vi "unflattenTemperatureAbsFromXML_Array.vi"(8 "error in (no error)":errorcluster, 9 "temperatureAbsUnitInXML":T1, 10 "xmlString":string, 11 "temperatureAbsForType":dbl[unit][](array[numeric])=[273.41179938779914, 273.6735987755983, 273.93539816339745, 274.19719755119655]) -> (0 "error out":errorcluster, 3 "temperatureAbs":dbl[unit][](array[numeric]))   [LabVIEW 2012, in "UnitsAndXML.lvlib"]
uses:
  <userlib>/Common/UnitsAndXML/UnitsAndXML.lvlib
  <userlib>/Common/UnitsAndXML/FlattenItemWithUnitToXML/FlattenTemperatureAbsToXML/TemperatureAbsUnit.ctl
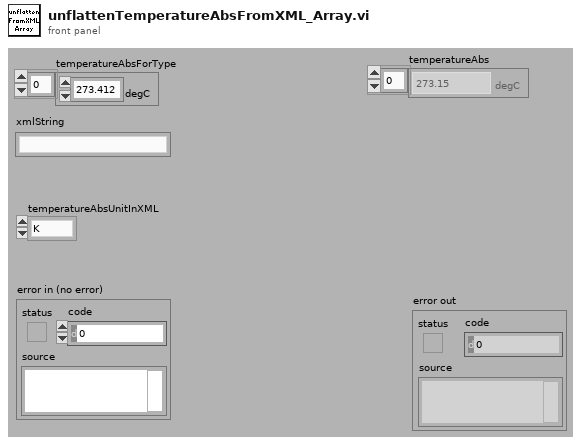
[diagram p1: front panel]
types:
  T1 = typedef "UnitsAndXML.lvlib/TemperatureAbsUnit.ctl" = enum16{"K", "degC", "degF"}
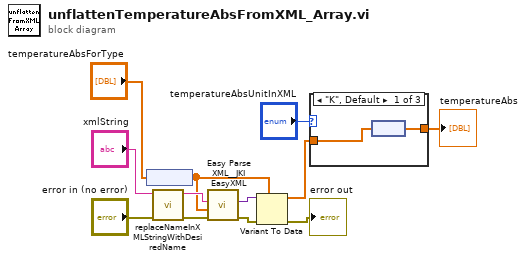
[diagram p0: block diagram]
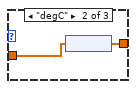
[diagram p2: hidden frame]
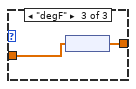
[diagram p3: hidden frame]
diagram:
  n1 = node("temperatureAbsForType") -> (w8:dbl[])
  n2 = call <userlib>:"replaceNameInXMLStringWithDesiredName.vi"("error in"="error in (no error)", "xmlString"="xmlString") -> ("error out"=w1:errorcluster, "revisedXMLString"=w9:string)  [unwired: 8 in]
  n3 = call <vilib>:"Easy Parse XML__JKI EasyXML.vi"("error in (no error)"=w1, "LabVIEW Data (Type)"=w8, "XML String"=w9) -> ("error out"=w4:errorcluster, "LabVIEW Data"=w11:variant)  [unwired: 7 in]
  n4 = Variant To Data(error in=w4, type=w8, Variant=w11) -> (data=w7:dbl[], error out=→"error out":errorcluster)
  n5 = case shown="\"K\", Default" "temperatureAbsUnitInXML" {
    tunnel: w7 -> [w13 w16 w18]
    tunnel: [w14 w15 w17] -> w6
    frame "K", Default {
      n6 = node(w13) -> (w14:dbl[unit][])
    }
    frame "degC" {
      n7 = node(w16) -> (w15:dbl[unit][])
    }
    frame "degF" {
      n8 = node(w18) -> (w17:dbl[unit][])
    }
  }
  "temperatureAbs" <- w6
